vi "Add Client Handler.vi"(8 "error in (no error)":errorcluster, 9 "Websocket Client Handler MTQ":refnum<class "Message Transport Queue.lvclass">, 10 "GUID":string, 11 "Websocket Server in":refnum<class "Websocket Server.lvclass">) -> (0 "error out":errorcluster, 3 "Websocket Server out":refnum<class "Websocket Server.lvclass">)   [LabVIEW 2016, in "Stream Mediator.lvlib" / "Websocket Server.lvclass"]
uses:
  <userlib>/Composed Systems/Stream/Mediator/Classes/Websocket Server Actor/Websocket Server/Websocket Server.lvclass
  <userlib>/Composed Systems/Stream/Mediator/Classes/Message Transport Queue/Message Transport Queue.lvclass
  C:/Program Files (x86)/National Instruments/LabVIEW 2016/user.lib/Composed Systems/Stream/Mediator/Classes/Message Transport Interface/Message Transport Interface.lvclass
  <userlib>/Composed Systems/Stream/Mediator/Classes/Websocket Server Actor/Websocket Server/Websocket Server.lvclass/Websocket Server.ctl
  <userlib>/Composed Systems/Stream/Mediator/Classes/Subscriber Look Up Table/Subscriber Look Up Table.lvclass
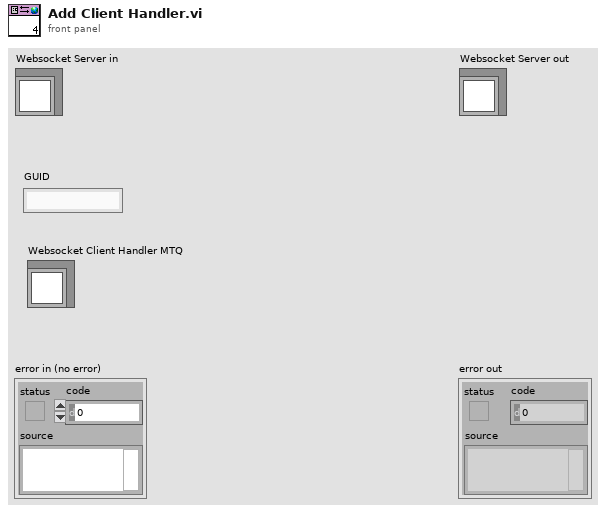
[diagram p1: front panel]
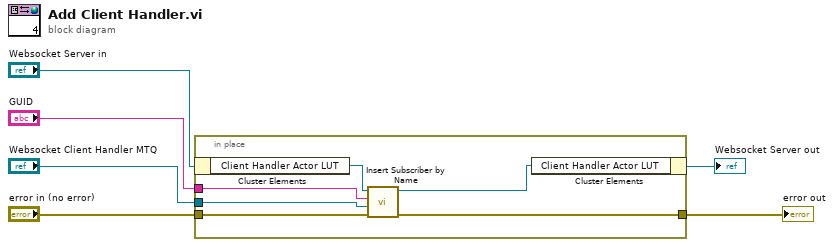
[diagram p0: block diagram]
diagram:
  n1 = in-place {
    in-place-border: "GUID" -> [w10]
    in-place-border: "Websocket Client Handler MTQ" -> [w9]
    in-place-border: "error in (no error)" -> [w8]
    in-place-border: [w7] -> w1
    n2 = in-place-cluster #1("Websocket Server in") -> ("Client Handler Actor LUT"=w12:refnum<class "Subscriber Look Up Table.lvclass">)
    n3 = call <userlib>:"Insert Subscriber by Name.vi"("error in (no error)"=w8, "Subscriber"=w9, "Topic Name"=w10, "Subscriber Index Look Up Table in"=w12) -> ("error out"=w7:errorcluster, "Subscriber Index Look Up Table out"=w11:refnum<class "Subscriber Look Up Table.lvclass">)  [unwired: 5 in, 1 out]
    n4 = in-place-cluster #1("Client Handler Actor LUT"=w11) -> (→"Websocket Server out":refnum<class "Websocket Server.lvclass">)
  }
  "error out" <- w1
